vi "Test Add Node To Dictionary.vi"(8 "error in (no error)":errorcluster) -> (0 "error out":errorcluster)   [LabVIEW 2017, in "Unit Tests.lvlib"]
uses:
  Unit Tests.lvlib
  source/Browser Core/Server Classes/Base Tree/Base Tree.lvclass
  source/Browser Core/Node Classes/Generic Node/Generic Node.lvclass
  source/Browser Core/Node Classes/Generic Node/Generic Node.lvclass/Generic Node.ctl
  source/Browser Core/Server Classes/Base Tree/Base Tree.lvclass/Base Tree.ctl
  <vilib>/addons/_JKI Toolkits/Caraya/classes/Test/Test.lvclass
  <vilib>/addons/_JKI Toolkits/Caraya/classes/Assert/Assert.lvclass
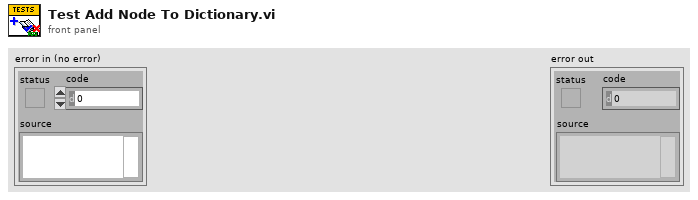
[diagram p1: front panel]
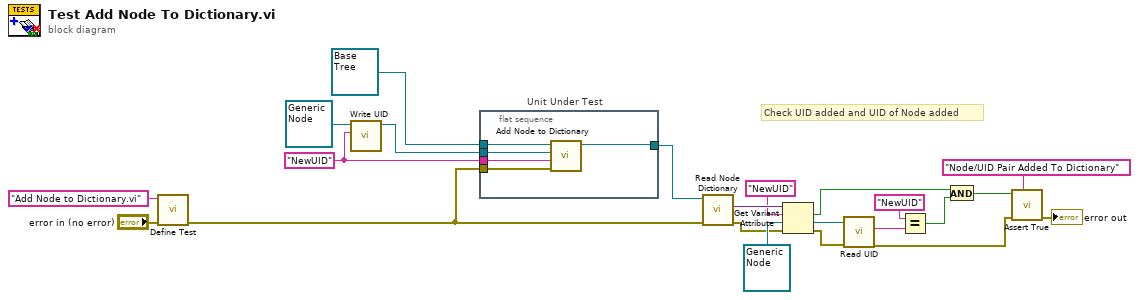
[diagram p0: block diagram]
diagram:
  w14 = "NewUID" ("UID")
  # "Check UID added and UID of Node added"
  n1 = call <vilib>:"Define Test.vi"("error in (no error)"="error in (no error)", "Label (VI Title)"="Add Node to Dictionary.vi") -> ("error out"=w13:errorcluster)  [unwired: 9 in]
  n2 = call "Write UID.vi"("UID"=w14, "Generic Node in"=refnum<class "Generic Node.lvclass"> refnum ("New Node")) -> ("Generic Node out"=w15:refnum<class "Generic Node.lvclass">)  [unwired: 8 in, 1 out]
  n3 = flat-sequence "Unit Under Test" {
    tunnel: w13 -> [w27]
    tunnel: refnum<class "Base Tree.lvclass"> refnum ("Base Tree in") -> [w26]
    tunnel: w15 -> [w25]
    tunnel: w14 -> [w24]
    tunnel: [w23] -> w12
    frame #0 {
      n4 = call "Add Node to Dictionary.vi"("Error In"=w27, "UID"=w24, "New Node"=w25, "Base Tree in"=w26) -> ("Base Tree out"=w23:refnum<class "Base Tree.lvclass">)  [unwired: 7 in]
    }
  }
  n5 = call "Read Node Dictionary.vi"("error in (no error)"=w13, "Base Tree in"=w12) -> ("error out"=w8:errorcluster, "Node Dictionary"=w11:variant)  [unwired: 7 in, 1 out]
  n6 = Get Variant Attribute(Variant=w11, name="NewUID" ("UID"), default value (empty Variant)=refnum<class "Generic Node.lvclass"> refnum ("New Node"), error in=w8) -> (found=w3:bool, value=w7:refnum<class "Generic Node.lvclass">, error out=w6:errorcluster)  [unwired: 1 out]
  n7 = call "Read UID.vi"("error in (no error)"=w6, "Generic Node in"=w7) -> ("error out"=w1:errorcluster, "UID"=w5:string)  [unwired: 7 in, 1 out]
  n8 = Equal?(x="NewUID" ("UID"), y=w5) -> (x = y?=w2:bool)
  n9 = And(x=w3, y=w2) -> (x .and. y?=w17:bool)
  n10 = call <vilib>:"Assert True.vi"("Label"="Node/UID Pair Added To Dictionary", "error in (no error)"=w1, "True?"=w17) -> ("error out"=→"error out":errorcluster)  [unwired: 8 in]
